vi "Example_template.vi"() -> ()   [LabVIEW 2015]
panel:
  out "error out":errorcluster
  out "function return 2":string
  # "hello_world.xlsx"
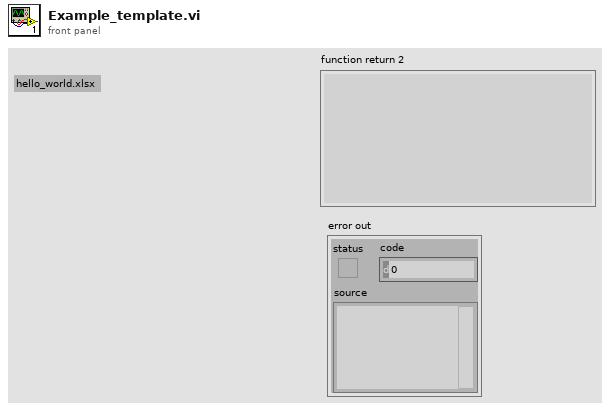
[diagram p1: front panel]
types:
  T1 = enum32{"invalid app kind", "Development System", "Run Time System", "Student Edition", "Embedded LabVIEW", "Evaluation", "Custom"}
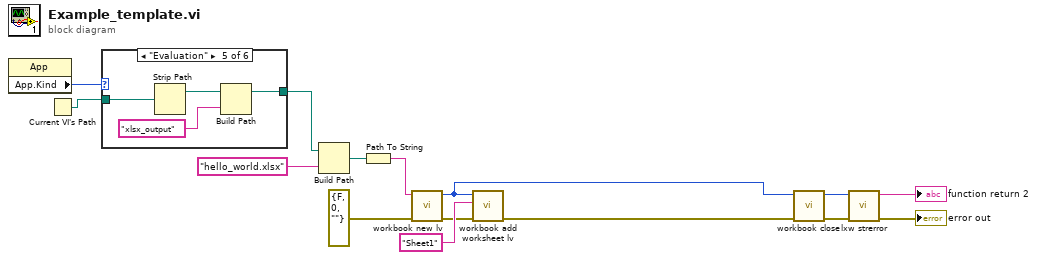
[diagram p0: block diagram]
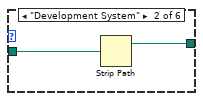
[diagram p3: hidden frame]
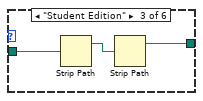
[diagram p4: hidden frame]
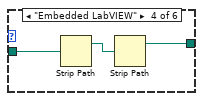
[diagram p5: hidden frame]
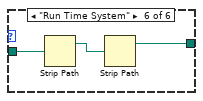
[diagram p6: hidden frame]
diagram:
  n1 = property class="App"() -> ("App.Kind"=w15:T1)  [unwired: 2 in, 2 out]
  n2 = Current VI's Path() -> (path=w14:path)
  n3 = case shown="\"Evaluation\"" w15 {
    tunnel: w14 -> [w16 w18 w21 w24 w28 w31]
    tunnel: [w16 w17 w19 w22 w26 w29] -> w13
    frame "invalid app kind", Default {
    }
    frame "Development System" {
      n4 = Strip Path(path=w18) -> (stripped path=w17:path)  [unwired: 1 out]
    }
    frame "Student Edition" {
      n5 = Strip Path(path=w21) -> (stripped path=w20:path)  [unwired: 1 out]
      n6 = Strip Path(path=w20) -> (stripped path=w19:path)  [unwired: 1 out]
    }
    frame "Embedded LabVIEW" {
      n7 = Strip Path(path=w24) -> (stripped path=w23:path)  [unwired: 1 out]
      n8 = Strip Path(path=w23) -> (stripped path=w22:path)  [unwired: 1 out]
    }
    frame "Evaluation" {
      n9 = Strip Path(path=w28) -> (stripped path=w27:path)  [unwired: 1 out]
      n10 = Build Path(base path=w27, name or relative path="xlsx_output") -> (appended path=w26:path)
    }
    frame "Run Time System" {
      n11 = Strip Path(path=w31) -> (stripped path=w30:path)  [unwired: 1 out]
      n12 = Strip Path(path=w30) -> (stripped path=w29:path)  [unwired: 1 out]
    }
  }
  n13 = Build Path(base path=w13, name or relative path="hello_world.xlsx" ("filename")) -> (appended path=w3:path)
  n14 = Path To String(path=w3) -> (string=w2:string)
  n15 = call "workbook new lv.vi"("error in (no error)"=errorcluster {"status"=FALSE, "code"=0, "source"=""}, "filename"=w2) -> ("error out"=w10:errorcluster, "function return"=w4:u32)  [unwired: 8 in]
  n16 = call "workbook add worksheet lv.vi"("error in (no error)"=w10, "sheetname"="Sheet1", "workbook"=w4) -> ("error out"=w1:errorcluster)  [unwired: 7 in, 1 out]
  n17 = call "workbook close.vi"("error in (no error)"=w1, "workbook"=w4) -> ("error out"=w6:errorcluster, "function return"=w8:u32)  [unwired: 8 in]
  n18 = call "lxw strerror.vi"("error in (no error)"=w6, "error_num"=w8) -> ("error out"=→"error out":errorcluster, "function return"=→"function return 2":string)  [unwired: 8 in]
